vi "2Pixel.vi"() -> ()   [LabVIEW 2009, in "menu item.lvclass"]
uses:
  menu item.lvclass
panel:
  out "2 pixel":u32
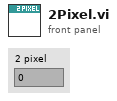
[diagram p1: front panel]
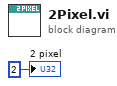
[diagram p0: block diagram]
diagram:
  "2 pixel" <- u32 2 ("1 pixel")
